vi "Corr Panel.vi"(8 "error in":errorcluster, 10 "adc session":T1={"niScope"={"channel cfg"=[], "sessions"=[], "multi cards"=FALSE, "channels"=0, "type"=enum."n/a", "memory [B/chn]"=0, "ext. clock [Hz]"=0.0, "samples count"=0, "use streaming"=FALSE, "proc setup"={"packet size [smpl]"=0, "current timeout [s]"=0.0, "blk2blk timeout [s]"=0.0, "event time"=timestamp(0 s since 1904-01-01), "temp sampl T [s]"=0.0, "data queue"=refnum, "stop notifier"=refnum, "proc ref"=refnum}, "sample width [B]"=0, "ranges [V]"=[], "trigger setup"={"coupling"=1, "level [V]"=0.0, "slope"=0, "mode"=enum."Immediate"}, "fs [Hz]"=0.0, "bitres [bit]"=0}, "3458A"={"channels"=[], "sync unit"={"VISA"="", "type"=enum."Picotest U6200A"}, "awg unit"={"type"=enum."Agilent 331xxA to 332xxA", "VISA"="", "enable 10MHz ref"=FALSE}, "sync mode"=enum."MASTER-SLAVE, MASTER clocked by TIMER", "streaming mode"=FALSE, "idn mode"=enum."Auto", "sampling mode"=enum."DCV", "Ts [s]"=0.0, "sample memory [B]"=0, "proc setup"={"channel id"=0, "packet size [smpl]"=0, "current timeout [s]"=0.0, "blk2blk timeout [s]"=0.0, "event time"=timestamp(0 s since 1904-01-01), "stop notifier"=refnum, "data queues"=[], "proc refs"=[], "bus semaphore"=refnum}, "sample size [B]"=0, "sample count"=0, "aux data"={"channel id"=0, "valid?"=[], "gain [V]"=[], "timestamp [s]"=[], "Ts [s]"=0.0, "abs timestamp"=timestamp(0 s since 1904-01-01), "t [deg C]"=[]}, "ranges [V]"=[], "aperture [s]"=0.0, "LEVEL trigger"={"edge"=enum."POS", "level [V]"=0.0, "coupling"=enum."DC"}, "trigger mode"=enum."AUTO", "measure temp.?"=FALSE, "disp mesages"=[], "shared bus?"=FALSE, "disable display?"=FALSE, "aper mode"=enum."Manual", "aper rules"=[]}, "dsdll"={"dsdll"={"dsdll path"=path "", "dsdll handle"=[], "output devices"=[], "capture devices"=[]}, "channels"=0, "device id"=0, "channel idns"=[], "proc setup"={"packet size [smpl]"=0, "current timeout [s]"=0.0, "blk2blk timeout [s]"=0.0, "event time"=timestamp(0 s since 1904-01-01), "data queue"=refnum, "stop notifier"=refnum, "proc ref"=refnum}, "samples count"=0, "fs [Hz]"=0.0}, "type"=enum."niScope", "channel idn str"=[], "aux instr idn str"=[], "modified?"=FALSE, "simadc"={"channels"=[], "range [V]"=0.0, "Ts step [s]"=0.0, "time [s]"=0.0, "fs [Hz]"=0.0, "count"=0, "smpl offset"=0, "set count"=0, "bit res"=0}, "force rst?"=FALSE, "exit mode"=enum."Immediate reset", "exit dly"=0.0, "exit tmr"=timestamp(0 s since 1904-01-01), "busy?"=FALSE, "accessed?"=FALSE, "QuADC session"={"channel cfg"=[], "sessions"=[], "multi cards"=FALSE, "channels"=0, "type"=enum."n/a", "memory [B/chn]"=0, "ext. clock [Hz]"=0.0, "samples count"=0, "use streaming"=FALSE, "proc setup"={"packet size [smpl]"=0, "current timeout [s]"=0.0, "blk2blk timeout [s]"=0.0, "event time"=timestamp(0 s since 1904-01-01), "temp sampl T [s]"=0.0, "data queue"=refnum, "stop notifier"=refnum, "proc ref"=refnum}, "sample width [B]"=0, "ranges [V]"=[], "trigger setup"={"coupling"=1, "level [V]"=0.0, "slope"=0, "mode"=enum."Immediate"}, "fs [Hz]"=0.0, "bitres [bit]"=0}} {"QuADC session"."trigger setup"."level [V]" format="%.2f"; "QuADC session"."trigger setup"."coupling" items=["AC"=0, "DC"=1, "HF Reject"=3, "LF Reject"=4, "AC Plus HF Reject"=1001]; "QuADC session"."channel cfg"."Clock fr. (Hz)" min=0.0 format="%#_9p"; "QuADC session"."channel cfg"."Number of JJ" min=1; "QuADC session"."channel cfg"."Range [Vpk]" min=0.0; "QuADC session"."channel cfg"."Channel" min=0; "3458A"."channels"."Range [Vpk]" min=0.0; "niScope"."trigger setup"."level [V]" format="%.2f"; "niScope"."trigger setup"."coupling" items=["AC"=0, "DC"=1, "HF Reject"=3, "LF Reject"=4, "AC Plus HF Reject"=1001]; "niScope"."channel cfg"."Range [Vpk]" min=0.0; "niScope"."channel cfg"."Channel" min=0}, 11 "transducers in":T45 {"transducers"."channels"."Phase index" min=1 step=1}) -> (0 "error out":errorcluster, 2 "adc session out":T1={"niScope"={"channel cfg"=[], "sessions"=[], "multi cards"=FALSE, "channels"=0, "type"=enum."n/a", "memory [B/chn]"=0, "ext. clock [Hz]"=0.0, "samples count"=0, "use streaming"=FALSE, "proc setup"={"packet size [smpl]"=0, "current timeout [s]"=0.0, "blk2blk timeout [s]"=0.0, "event time"=timestamp(0 s since 1904-01-01), "temp sampl T [s]"=0.0, "data queue"=refnum, "stop notifier"=refnum, "proc ref"=refnum}, "sample width [B]"=0, "ranges [V]"=[], "trigger setup"={"coupling"=1, "level [V]"=0.0, "slope"=0, "mode"=enum."Immediate"}, "fs [Hz]"=0.0, "bitres [bit]"=0}, "3458A"={"channels"=[], "sync unit"={"VISA"="", "type"=enum."Picotest U6200A"}, "awg unit"={"type"=enum."Agilent 331xxA to 332xxA", "VISA"="", "enable 10MHz ref"=FALSE}, "sync mode"=enum."MASTER-SLAVE, MASTER clocked by TIMER", "streaming mode"=FALSE, "idn mode"=enum."Auto", "sampling mode"=enum."DCV", "Ts [s]"=0.0, "sample memory [B]"=0, "proc setup"={"channel id"=0, "packet size [smpl]"=0, "current timeout [s]"=0.0, "blk2blk timeout [s]"=0.0, "event time"=timestamp(0 s since 1904-01-01), "stop notifier"=refnum, "data queues"=[], "proc refs"=[], "bus semaphore"=refnum}, "sample size [B]"=0, "sample count"=0, "aux data"={"channel id"=0, "valid?"=[], "gain [V]"=[], "timestamp [s]"=[], "Ts [s]"=0.0, "abs timestamp"=timestamp(0 s since 1904-01-01), "t [deg C]"=[]}, "ranges [V]"=[], "aperture [s]"=0.0, "LEVEL trigger"={"edge"=enum."POS", "level [V]"=0.0, "coupling"=enum."DC"}, "trigger mode"=enum."AUTO", "measure temp.?"=FALSE, "disp mesages"=[], "shared bus?"=FALSE, "disable display?"=FALSE, "aper mode"=enum."Manual", "aper rules"=[]}, "dsdll"={"dsdll"={"dsdll path"=path "", "dsdll handle"=[], "output devices"=[], "capture devices"=[]}, "channels"=0, "device id"=0, "channel idns"=[], "proc setup"={"packet size [smpl]"=0, "current timeout [s]"=0.0, "blk2blk timeout [s]"=0.0, "event time"=timestamp(0 s since 1904-01-01), "data queue"=refnum, "stop notifier"=refnum, "proc ref"=refnum}, "samples count"=0, "fs [Hz]"=0.0}, "type"=enum."niScope", "channel idn str"=[], "aux instr idn str"=[], "modified?"=FALSE, "simadc"={"channels"=[], "range [V]"=0.0, "Ts step [s]"=0.0, "time [s]"=0.0, "fs [Hz]"=0.0, "count"=0, "smpl offset"=0, "set count"=0, "bit res"=0}, "force rst?"=FALSE, "exit mode"=enum."Immediate reset", "exit dly"=0.0, "exit tmr"=timestamp(0 s since 1904-01-01), "busy?"=FALSE, "accessed?"=FALSE, "QuADC session"={"channel cfg"=[], "sessions"=[], "multi cards"=FALSE, "channels"=0, "type"=enum."n/a", "memory [B/chn]"=0, "ext. clock [Hz]"=0.0, "samples count"=0, "use streaming"=FALSE, "proc setup"={"packet size [smpl]"=0, "current timeout [s]"=0.0, "blk2blk timeout [s]"=0.0, "event time"=timestamp(0 s since 1904-01-01), "temp sampl T [s]"=0.0, "data queue"=refnum, "stop notifier"=refnum, "proc ref"=refnum}, "sample width [B]"=0, "ranges [V]"=[], "trigger setup"={"coupling"=1, "level [V]"=0.0, "slope"=0, "mode"=enum."Immediate"}, "fs [Hz]"=0.0, "bitres [bit]"=0}} {"QuADC session"."trigger setup"."level [V]" format="%.2f"; "QuADC session"."trigger setup"."coupling" items=["AC"=0, "DC"=1, "HF Reject"=3, "LF Reject"=4, "AC Plus HF Reject"=1001]; "QuADC session"."channel cfg"."Clock fr. (Hz)" min=0.0 format="%#_9p"; "QuADC session"."channel cfg"."Number of JJ" min=1; "QuADC session"."channel cfg"."Range [Vpk]" min=0.0; "QuADC session"."channel cfg"."Channel" min=0; "3458A"."channels"."Range [Vpk]" min=0.0; "niScope"."trigger setup"."level [V]" format="%.2f"; "niScope"."trigger setup"."coupling" items=["AC"=0, "DC"=1, "HF Reject"=3, "LF Reject"=4, "AC Plus HF Reject"=1001]; "niScope"."channel cfg"."Range [Vpk]" min=0.0; "niScope"."channel cfg"."Channel" min=0}, 3 "transducers out":T45 {"transducers"."channels"."Phase index" min=1 step=1})   [LabVIEW 2018]
doc: "Configuration panel for corrections."
uses:
  Corr Setup.ctl
  Corr Tranducer Item.ctl
  Corr Digitizers.ctl
  Corr Digitizer Channel.ctl
  adc/ADC Session.ctl
  drivers/niScope/niScope Session.ctl
  drivers/niScope/niScope Virtual Channel Config.ctl
  drivers/niScope/niScope Virtual Channel Mode.ctl
  drivers/niScope/niScope Virtual Channel Input Z.ctl
  drivers/niScope/niScope Virtual Channel Coupling.ctl
  drivers/niScope/niScope Type.ctl
  drivers/niScope/niScope Digitizing Process Options.ctl
  drivers/niScope/niScope Data Packet.ctl
  drivers/niScope/niScope Trigger Setup.ctl
  <instrlib>/niScope/Controls/niScope trigger coupling.ctl
  <instrlib>/niScope/Controls/niScope trigger slope.ctl
  drivers/DMM/3458A Digitizer Session.ctl
  drivers/DMM/3458A Virtual Channel Config.ctl
  drivers/Counter/Counter Session.ctl
  drivers/Counter/Counter Type.ctl
  drivers/AWG/AWG Session.ctl
  drivers/AWG/AWG Type.ctl
  drivers/DMM/3458A Sync Mode.ctl
  drivers/DMM/3458A Idn Mode.ctl
  drivers/DMM/3458A Digitizing Low Levels/Configure/Sampling Mode.ctl
  drivers/DMM/3458A Digitizing Process Options.ctl
  drivers/DMM/3458A Data Packet.ctl
  drivers/DMM/3458A Aux Record Data.ctl
  drivers/DMM/3458A Digitizing Low Levels/Configure/Level Setup.ctl
  drivers/DMM/3458A Digitizing Low Levels/Configure/First Sample Trigger.ctl
  drivers/DMM/3458A Aperture Selection Mode.ctl
  drivers/dsdll/DSDLL Session.ctl
  drivers/dsdll/dsdll source distribution/dsdll_instance.ctl
  drivers/dsdll/dsdll source distribution/dsdll_device_record.ctl
  drivers/dsdll/DSDLL Process Config.ctl
  drivers/dsdll/DSDLL Data Packet.ctl
  adc/ADC Type.ctl
  drivers/simulated_adc/SimAdc Config.ctl
  drivers/simulated_adc/SimAdc Channel Cfg.ctl
  adc/ADC On Close Action.ctl
  drivers/Quatsch_driver/QuADCDriver/QuADC Session.ctl
  drivers/Quatsch_driver/QuADCDriver/QuADC Virtual Channel Config.ctl
  drivers/Quatsch_driver/QuADCDriver/QuADC Virtual Channel Mode.ctl
  drivers/Quatsch_driver/QuADCDriver/QuADC Virtual Channel Input Z.ctl
  drivers/Quatsch_driver/QuADCDriver/QuADC Virtual Channel Coupling.ctl
  drivers/Quatsch_driver/QuADCDriver/QuADC Type.ctl
  drivers/Quatsch_driver/QuADCDriver/QuADC Digitizing Process Options.ctl
  drivers/Quatsch_driver/QuADCDriver/QuADC Data Packet.ctl
  drivers/Quatsch_driver/QuADCDriver/QuADC Trigger Setup.ctl
  varilib/SGUI Assign References Mode.ctl
  other/GUI Panel Control Action.ctl
  varilib/SGUI Assign Multiple Strings With Tags By Label.vi
  varilib/varilib.lvlib
  drivers/niScope/niScope Virtual Digitizer.lvlib
  drivers/DMM/3458A Virtual Digitizer.lvlib
  drivers/Counter/Counter.lvlib
  drivers/AWG/AWG.lvlib
  drivers/DMM/3458A Digitizing Low Levels/3458A Digitizing Low Levels.lvlib
  drivers/dsdll/DSDLL Virtual Digitizer.lvlib
  drivers/Quatsch_driver/QuADCDriver/QuADC Virtual Digitizer.lvlib
  drivers/dsdll/dsdll source distribution/dsdll.lvlib
panel:
  in  "tc corr":enum32{"Transducers", "Digitizers"}(tab)
  in  "trans list":T43(array[cluster]) caption="List of the transducers" {"Phase index" min=1 step=1; "chn lo" items=["Not used"]}
  out "dig corr stat":string caption="Correction status"
  in  "btn check dig":bool
  in  "btn reload dig":bool
  in  "btn clear dig":bool
  out "dig corr chns":T44[](array[typedef]) caption="Correction channels"
  out "dig corr path":string caption="Correction file path"
  out "dig corr name":string caption="Correction name"
  in  "btn open dig":bool
  out "status":string caption="Status"
  in  "btn cancel":bool
  in  "btn ok":bool
  # "IP Address"
  # "."
  # "."
  # "."
  # ":"
  # "IP Address"
  # "."
  # "."
  # "."
  # ":"
  # "ADC:"
  # "ADC:"
  # "ADC:"
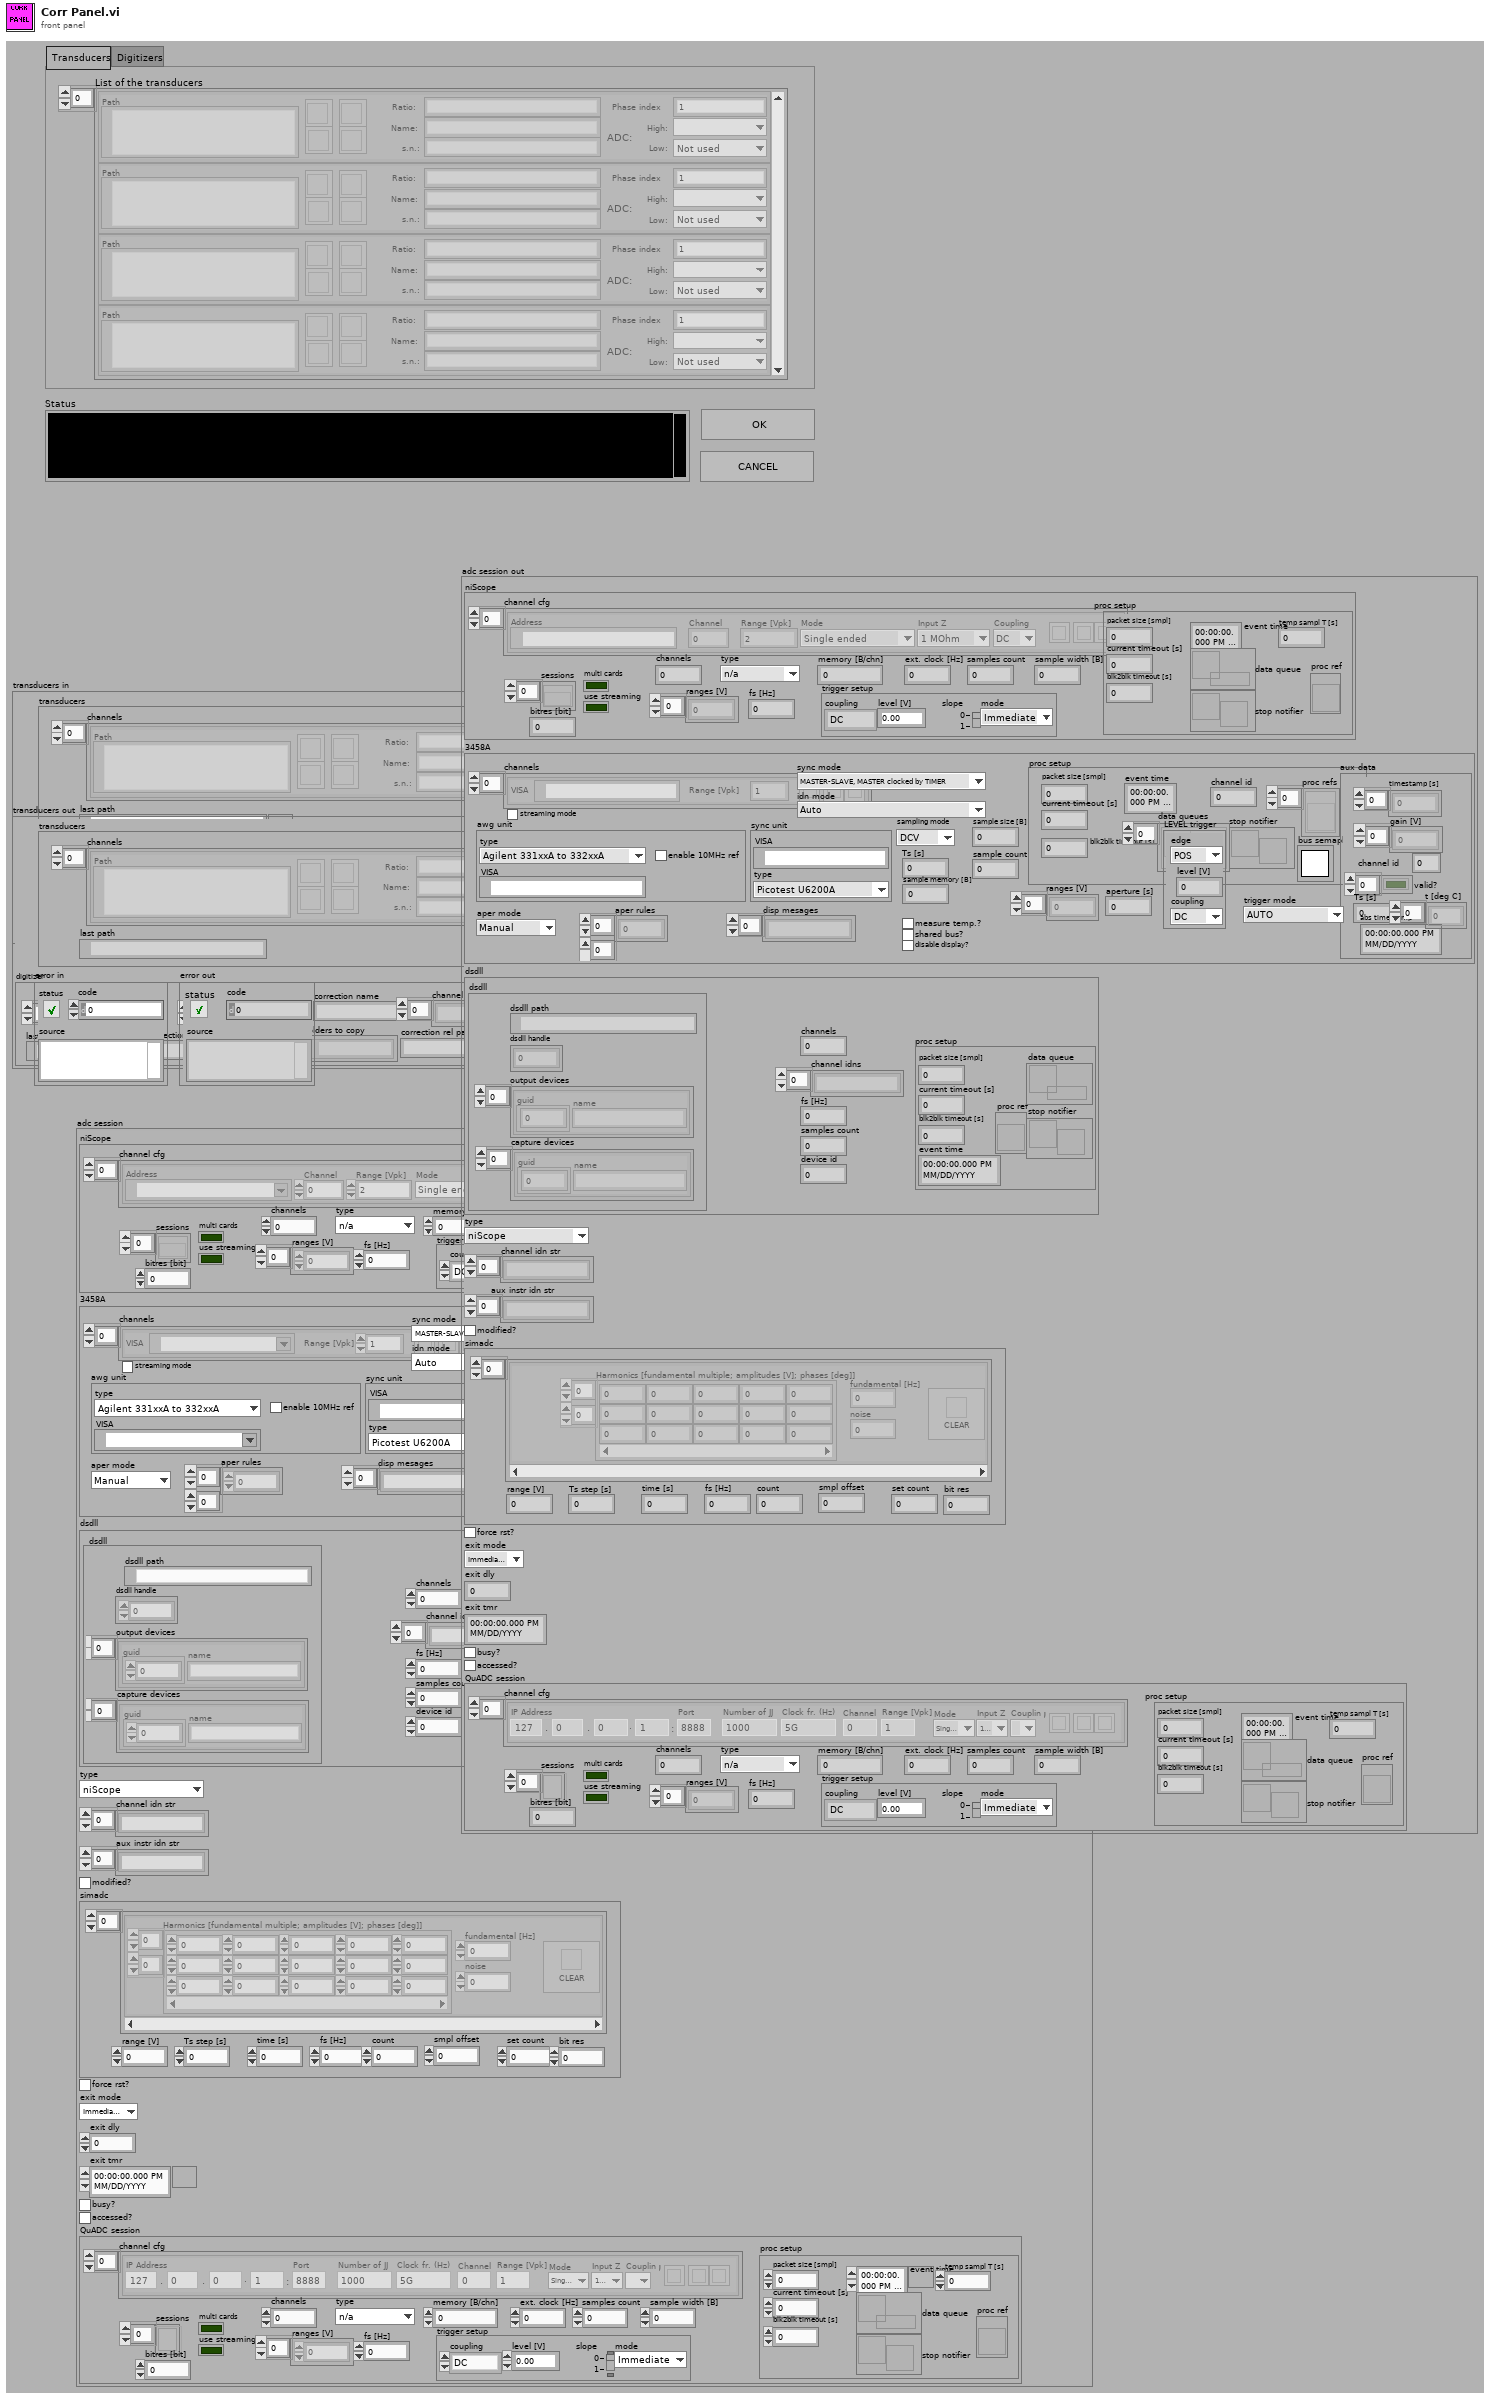
[diagram p1: front panel]
types:
  T1 = typedef "ADC Session.ctl" = cluster{"niScope":T2, "3458A":T12, "dsdll":T27, "type":T31, "channel idn str":string[], "aux instr idn str":string[], "modified?":bool, "simadc":T32, "force rst?":bool, "exit mode":T34, "exit dly":dbl, "exit tmr":timestamp, "busy?":bool, "accessed?":bool, "QuADC session":T35}
  T2 = typedef "niScope Virtual Digitizer.lvlib/niScope Session.ctl" = cluster{"channel cfg":T3[], "sessions":refnum<k20>[], "multi cards":bool, "channels":i32, "type":T7, "memory [B/chn]":i32, "ext. clock [Hz]":dbl, "samples count":i64, "use streaming":bool, "proc setup":T8, "sample width [B]":i32, "ranges [V]":dbl[], "trigger setup":T9, "fs [Hz]":dbl, "bitres [bit]":i32}
  T3 = typedef "niScope Virtual Digitizer.lvlib/niScope Virtual Channel Config.ctl" = cluster{"Address":refnum<k15>, "Channel":i32, "Mode":T4, "Input Z":T5, "Coupling":T6, "Range [Vpk]":dbl, "btn clr":bool, "btn up":bool, "btn down":bool}
  T4 = typedef "niScope Virtual Digitizer.lvlib/niScope Virtual Channel Mode.ctl" = enum16{"Single ended", "Unbal. differential", "Differential"}
  T5 = typedef "niScope Virtual Digitizer.lvlib/niScope Virtual Channel Input Z.ctl" = enum16{"1 MOhm", "50 Ohm"}
  T6 = typedef "niScope Virtual Digitizer.lvlib/niScope Virtual Channel Coupling.ctl" = enum16{"AC", "DC", "GND"}
  T7 = typedef "niScope Virtual Digitizer.lvlib/niScope Type.ctl" = enum16{"n/a", "5922"}
  T8 = typedef "niScope Virtual Digitizer.lvlib/niScope Digitizing Process Options.ctl" = cluster{"packet size [smpl]":i64, "current timeout [s]":dbl, "blk2blk timeout [s]":dbl, "event time":timestamp, "temp sampl T [s]":dbl, "data queue":refnum<queue>, "stop notifier":refnum<notifier>, "proc ref":refnum<vi>}
  T9 = typedef "niScope Virtual Digitizer.lvlib/niScope Trigger Setup.ctl" = cluster{"coupling":T10, "level [V]":dbl, "slope":T11, "mode":enum16{"Immediate", "External", "Level"}}
  T10 = typedef "niScope trigger coupling.ctl" = u16
  T11 = typedef "niScope trigger slope.ctl" = i32
  T12 = typedef "3458A Virtual Digitizer.lvlib/3458A Digitizer Session.ctl" = cluster{"channels":T13[], "sync unit":T14, "awg unit":T16, "sync mode":T18, "streaming mode":bool, "idn mode":T19, "sampling mode":T20, "Ts [s]":dbl, "sample memory [B]":i32, "proc setup":T21, "sample size [B]":i32, "sample count":i32, "aux data":T23, "ranges [V]":dbl[], "aperture [s]":dbl, "LEVEL trigger":T24, "trigger mode":T25, "measure temp.?":bool, "disp mesages":string[], "shared bus?":bool, "disable display?":bool, "aper mode":T26, "aper rules":dbl[][]}
  T13 = typedef "3458A Virtual Digitizer.lvlib/3458A Virtual Channel Config.ctl" = cluster{"VISA":refnum<visa-resource-name>, "Range [Vpk]":dbl, "btn clr":bool, "btn up":bool, "btn down":bool}
  T14 = typedef "Counter.lvlib/Counter Session.ctl" = cluster{"VISA":refnum<visa-resource-name>, "type":T15}
  T15 = typedef "Counter.lvlib/Counter Type.ctl" = enum16{"Picotest U6200A", "dummy"}
  T16 = typedef "AWG.lvlib/AWG Session.ctl" = cluster{"type":T17, "VISA":refnum<visa-resource-name>, "enable 10MHz ref":bool}
  T17 = typedef "AWG.lvlib/AWG Type.ctl" = enum16{"Agilent 331xxA to 332xxA", "Agilent 335xxA to 336xxA", "Tektronix AFG3101C", "dummy"}
  T18 = typedef "3458A Virtual Digitizer.lvlib/3458A Sync Mode.ctl" = enum16{"MASTER-SLAVE, MASTER clocked by TIMER", "MASTER-SLAVE, MASTER clocked by AWG", "ALL clocked by AWG", "MASTER-SLAVE, ALL clocked by TIMER", "ALL clocked by AWG with DFLL"}
  T19 = typedef "3458A Virtual Digitizer.lvlib/3458A Idn Mode.ctl" = enum16{"Auto", "Sequential (chn A, chn B, ...)", "From calibration string"}
  T20 = typedef "3458A Virtual Digitizer.lvlib/3458A Digitizing Low Levels.lvlib/Sampling Mode.ctl" = enum16{"DCV", "DSDC", "DSAC"}
  T21 = typedef "3458A Virtual Digitizer.lvlib/3458A Digitizing Process Options.ctl" = cluster{"channel id":i32, "packet size [smpl]":i32, "current timeout [s]":dbl, "blk2blk timeout [s]":dbl, "event time":timestamp, "stop notifier":refnum<notifier>, "data queues":refnum<queue>[], "proc refs":refnum<vi>[], "bus semaphore":T22}
  T22 = typedef "Semaphore RefNum" = refnum<k1>
  T23 = typedef "3458A Virtual Digitizer.lvlib/3458A Aux Record Data.ctl" = cluster{"channel id":i32, "valid?":bool[], "gain [V]":dbl[], "timestamp [s]":dbl[], "Ts [s]":dbl, "abs timestamp":timestamp, "t [deg C]":dbl[]}
  T24 = typedef "3458A Virtual Digitizer.lvlib/3458A Digitizing Low Levels.lvlib/Level Setup.ctl" = cluster{"edge":enum16{"POS", "NEG"}, "level [V]":dbl, "coupling":enum16{"DC", "AC"}}
  T25 = typedef "3458A Virtual Digitizer.lvlib/3458A Digitizing Low Levels.lvlib/First Sample Trigger.ctl" = enum16{"AUTO", "EXT", "SYN", "SGL", "HOLD", "LEVEL"}
  T26 = typedef "3458A Virtual Digitizer.lvlib/3458A Aperture Selection Mode.ctl" = enum16{"Manual", "Maximum", "Table"}
  T27 = typedef "DSDLL Virtual Digitizer.lvlib/DSDLL Session.ctl" = cluster{"dsdll":T28, "channels":i32, "device id":i32, "channel idns":string[], "proc setup":T30, "samples count":i32, "fs [Hz]":dbl}
  T28 = typedef "dsdll.lvlib/dsdll_instance.ctl" = cluster{"dsdll path":path, "dsdll handle":u8[], "output devices":T29[], "capture devices":T29[]}
  T29 = typedef "dsdll.lvlib/dsdll_device_record.ctl" = cluster{"guid":u8[], "name":string}
  T30 = typedef "DSDLL Virtual Digitizer.lvlib/DSDLL Process Config.ctl" = cluster{"packet size [smpl]":i32, "current timeout [s]":dbl, "blk2blk timeout [s]":dbl, "event time":timestamp, "data queue":refnum<queue>, "stop notifier":refnum<notifier>, "proc ref":refnum<vi>}
  T31 = typedef "ADC Type.ctl" = enum16{"niScope", "3458A", "DirectSound DLL", "dummy", "QuADC"}
  T32 = typedef "SimAdc Config.ctl" = cluster{"channels":T33[], "range [V]":dbl, "Ts step [s]":dbl, "time [s]":dbl, "fs [Hz]":dbl, "count":i64, "smpl offset":i64, "set count":i64, "bit res":i32}
  T33 = typedef "SimAdc Channel Cfg.ctl" = cluster{"harmonics":dbl[][], "btn clear":bool, "noise":dbl, "fundamental [Hz]":dbl}
  T34 = typedef "ADC On Close Action.ctl" = enum16{"Immediate reset", "Delayed reset"}
  T35 = typedef "QuADC Virtual Digitizer.lvlib/QuADC Session.ctl" = cluster{"channel cfg":T36[], "sessions":refnum<k5>[], "multi cards":bool, "channels":i32, "type":T40, "memory [B/chn]":i32, "ext. clock [Hz]":dbl, "samples count":i64, "use streaming":bool, "proc setup":T41, "sample width [B]":i32, "ranges [V]":dbl[], "trigger setup":T42, "fs [Hz]":dbl, "bitres [bit]":i32}
  T36 = typedef "QuADC Virtual Digitizer.lvlib/QuADC Virtual Channel Config.ctl" = cluster{"Channel":i32, "Mode":T37, "Input Z":T38, "Coupling":T39, "Range [Vpk]":dbl, "btn clr":bool, "btn up":bool, "btn down":bool, "IP address A":u8, "IP address B":u8, "IP address C":u8, "IP address D":u8, "Port":u16, "Number of JJ":u32, "Clock fr. (Hz)":dbl}
  T37 = typedef "QuADC Virtual Digitizer.lvlib/QuADC Virtual Channel Mode.ctl" = enum16{"Single ended", "Unbal. differential", "Differential"}
  T38 = typedef "QuADC Virtual Digitizer.lvlib/QuADC Virtual Channel Input Z.ctl" = enum16{"1 MOhm", "50 Ohm"}
  T39 = typedef "QuADC Virtual Digitizer.lvlib/QuADC Virtual Channel Coupling.ctl" = enum16{"AC", "DC", "GND"}
  T40 = typedef "QuADC Virtual Digitizer.lvlib/QuADC Type.ctl" = enum16{"n/a", "v1"}
  T41 = typedef "QuADC Virtual Digitizer.lvlib/QuADC Digitizing Process Options.ctl" = cluster{"packet size [smpl]":i64, "current timeout [s]":dbl, "blk2blk timeout [s]":dbl, "event time":timestamp, "temp sampl T [s]":dbl, "data queue":refnum<queue>, "stop notifier":refnum<notifier>, "proc ref":refnum<vi>}
  T42 = typedef "QuADC Virtual Digitizer.lvlib/QuADC Trigger Setup.ctl" = cluster{"coupling":T10, "level [V]":dbl, "slope":T11, "mode":enum16{"Immediate", "External", "Level"}}
  T43 = cluster{"Path":path, "Ratio:":string, "Name:":string, "btn rem":bool, "btn up":bool, "btn down":bool, "s.n.:":string, "btn open":bool, "ratio o/i":dbl, "chn hi":u16, "chn lo":u16, "Phase index":i32}[]
  T44 = typedef "Corr Digitizer Channel.ctl" = cluster{"Correction identifier":string, "Channel correction file ok?":bool, "Channel matches digitizer HW?":bool, "Correction channel name":string, "HW channel identifier":string}
  T45 = typedef "Corr Setup.ctl" = cluster{"transducers":cluster{"channels":T46[], "last path":path}, "digitizer":T47}
  T46 = typedef "Corr Tranducer Item.ctl" = cluster{"Path":path, "Ratio:":string, "Name:":string, "btn rem":bool, "btn up":bool, "btn down":bool, "s.n.:":string, "btn open":bool, "ratio o/i":dbl, "chn hi":u16, "chn lo":u16, "Phase index":i32}
  T47 = typedef "Corr Digitizers.ctl" = cluster{"last path":path, "channel paths":path[], "channel idns":string[], "correction name":string, "channel names":string[], "folders to copy":path[], "channel valid":bool[], "correction path":path, "correction rel path":string, "rel folders to copy":string[]}
  T48 = typedef "GUI Panel Control Action.ctl" = enum16{"Open panel", "Close panel", "Bring To Front"}
  T49 = typedef "varilib.lvlib/SGUI Assign References Mode.ctl" = enum16{"Add to stack", "Overwrite", "Release last", "Release ID"}
  T50 = cluster{"Path":path, "Ratio:":string, "Name:":string, "btn rem":bool, "btn up":bool, "btn down":bool, "s.n.:":string, "btn open":bool, "ratio o/i":dbl, "chn hi":u16, "chn lo":u16, "Phase index":i32}
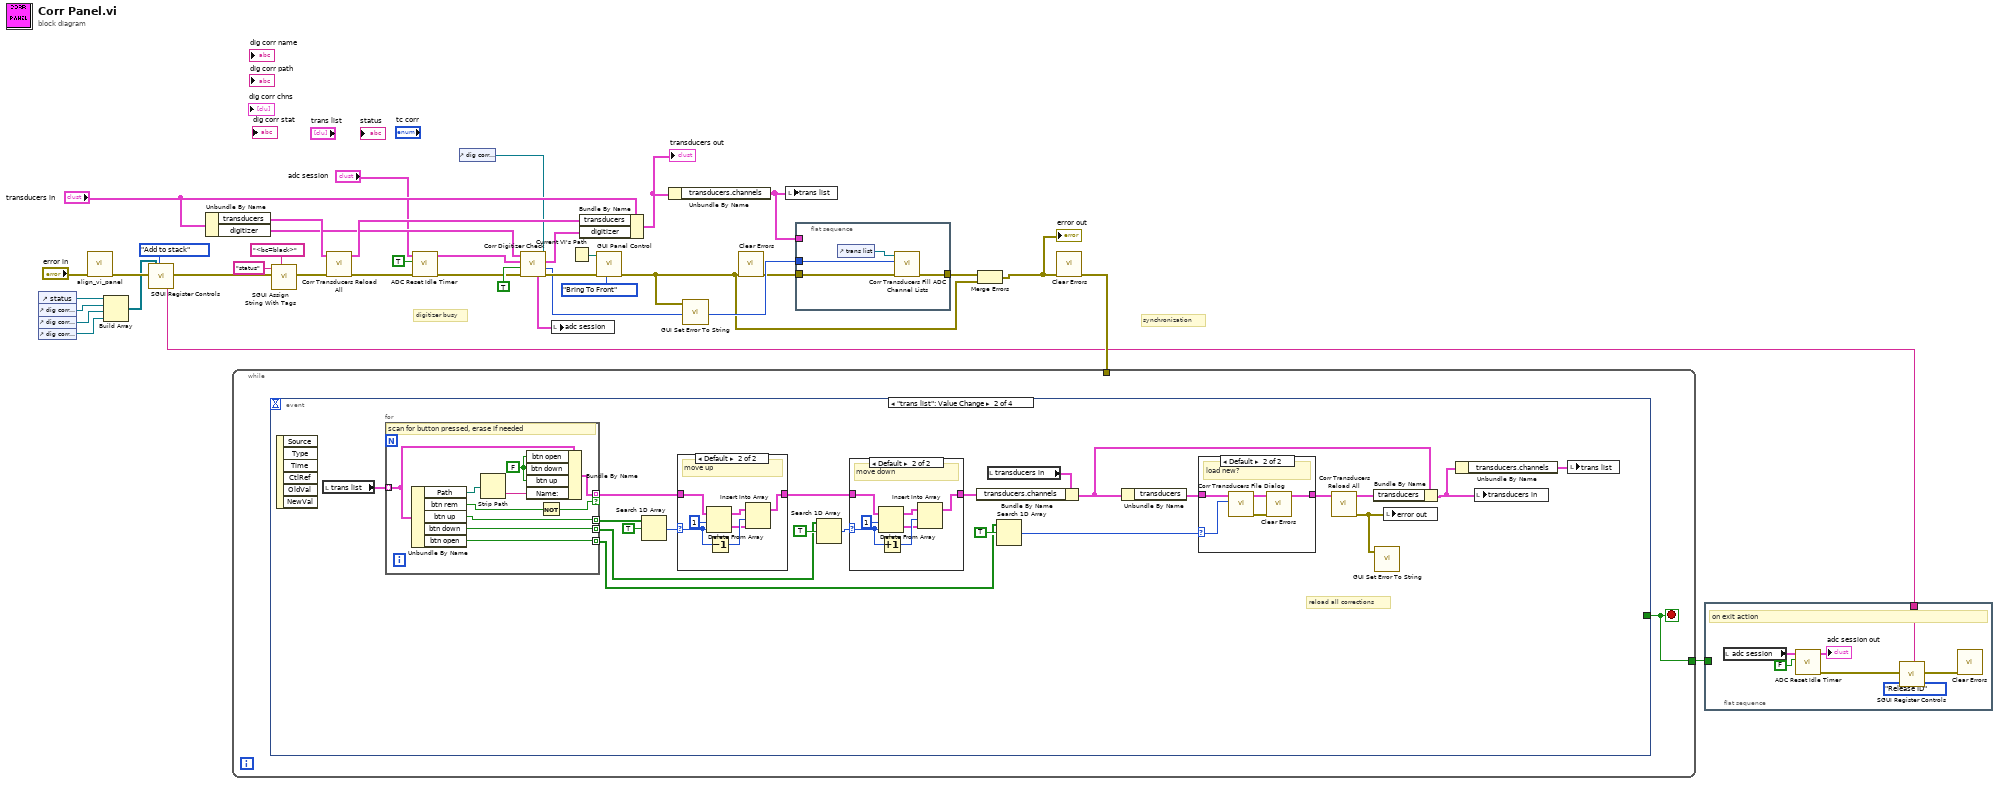
[diagram p0: block diagram]
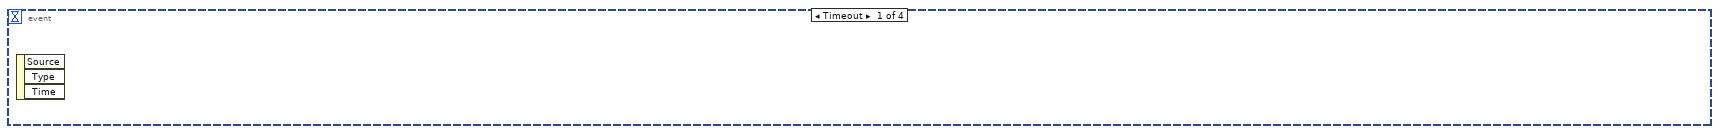
[diagram p2: hidden frame]
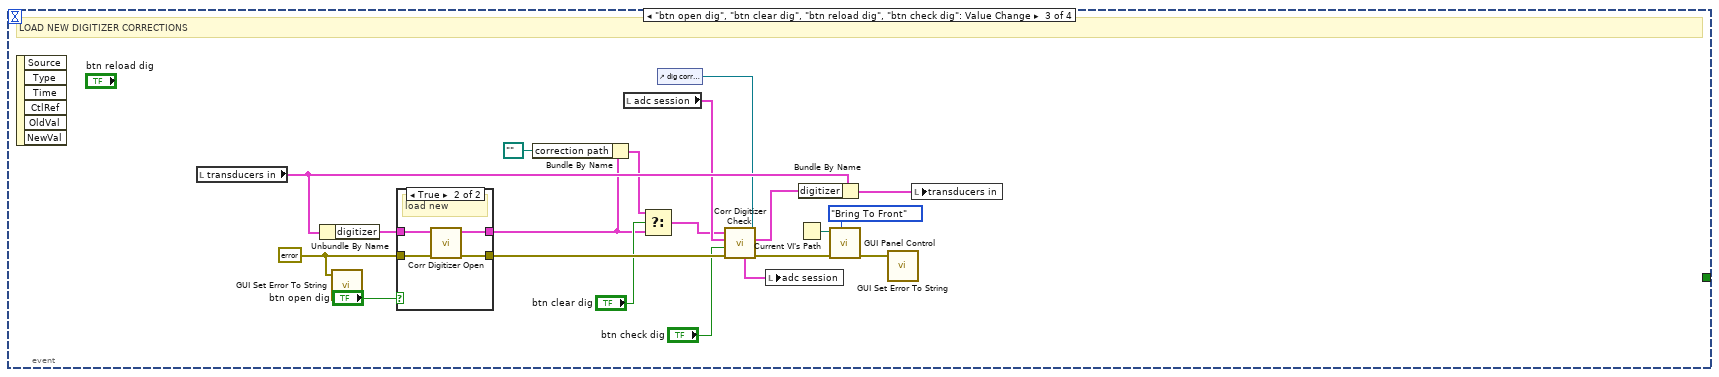
[diagram p6: hidden frame]
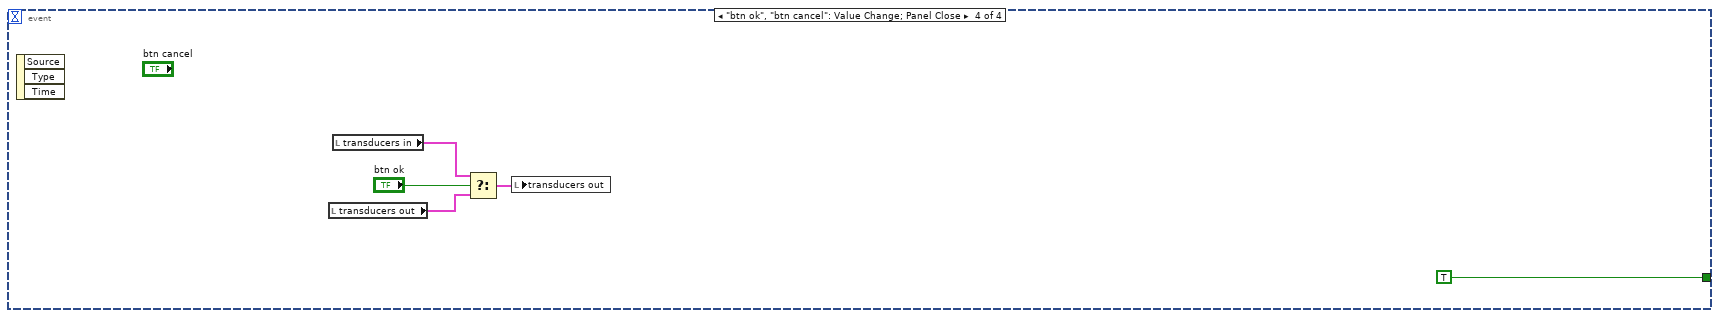
[diagram p8: hidden frame]
diagram:
  # "digitizer busy"
  # "synchronization"
  n1 = control-ref of="status"() -> (w24:refnum<vi>)
  n2 = control-ref of="dig corr name"() -> (w23:refnum<vi>)
  n3 = control-ref of="dig corr path"() -> (w22:refnum<vi>)
  n4 = control-ref of="dig corr stat"() -> (w21:refnum<vi>)
  n5 = call "align_vi_panel.vi"("error in"="error in") -> ("error out"=w38:errorcluster)  [unwired: 10 in]
  n6 = Build Array(w24, w23, w22, w21) -> (w25:refnum<vi>[])
  n7 = call "SGUI Register Controls.vi"("error in"=w38, "control references (empty)"=w25, "register mode (overwrite)"=SGUI_Assign_References_Mode."Add to stack") -> ("assigned ID"=w7:string, "error out"=w35:errorcluster)  [unwired: 14 in, 1 out]
  n8 = Unbundle By Name("transducers in") -> ("transducers"=w29:cluster{"channels":T46[], "last path":path}, "digitizer"=w19:T47)
  n9 = call-poly "SGUI Assign String With Tags.vi"("error in"=w35, "label(s) (empty)"="status", "string (empty)"="<bc=black>") -> ("error out"=w30:errorcluster)  [unwired: 7 in, 1 out]
  n10 = call "Corr Transducers Reload All.vi"("error in"=w30, "transducers in"=w29) -> ("error out"=w6:errorcluster, "transducers out"=w27:cluster{"channels":T46[], "last path":path})  [unwired: 8 in]
  n11 = call "ADC Reset Idle Timer.vi"("error in"=w6, "set busy (False)"=TRUE, "adc session in"="adc session") -> ("error out"=w4:errorcluster, "adc session out"=w2:T1)  [unwired: 7 in]
  n12 = control-ref of="dig corr chns"() -> (w17:refnum<vi>)
  n13 = call "Corr Digitizer Check.vi"("dig corr chns ref"=w17, "error in"=w4, "check HW? (False)"=TRUE, "adc session"=w2, "digitizer corrections in"=w19) -> ("error out"=w16:errorcluster, "adc chan. count"=w12:i32, "digitizer corrections out"=w20:T47, "adc session out"=w1:T1)  [unwired: 3 in]
  n14 = local write "adc session"(w1) -> ()
  n15 = Current VI's Path() -> (path=w15:path)
  n16 = Bundle By Name(cluster="transducers in", "transducers"=w27, "digitizer"=w20) -> (w26:T45)
  "transducers out" <- w26
  n17 = call "GUI Panel Control.vi"("action (open panel)"=GUI_Panel_Control_Action."Bring To Front", "error in (no error)"=w16, "vi path"=w15) -> ("error out"=w9:errorcluster)  [unwired: 8 in]
  n18 = Unbundle By Name(w26) -> ("transducers.channels"=w13:T46[])
  n19 = call "GUI Set Error To String.vi"("error in (no error)"=w9) -> ()  [unwired: 4 in]
  n20 = call <vilib>:"Clear Errors.vi"("error in (no error)"=w9) -> ("error out"=w11:errorcluster)  [unwired: 5 in, 1 out]
  n21 = local write "trans list"(w13) -> ()
  n22 = flat-sequence {
    tunnel: w11 -> [w42]
    tunnel: [w41] -> w10
    tunnel: w13 -> [_]
    tunnel: w12 -> [w40]
    frame #0 {
      n23 = control-ref of="trans list"() -> (w39:refnum<vi>)
      n24 = call "Corr Transducers Fill ADC Channel Lists.vi"("error in"=w42, "digitizer channels count (0)"=w40, "transducer list ref"=w39) -> ("error out"=w41:errorcluster)  [unwired: 7 in, 1 out]
    }
  }
  n25 = Merge Errors(w10, w9) -> (w8:errorcluster)
  "error out" <- w8
  n26 = call <vilib>:"Clear Errors.vi"("error in (no error)"=w8) -> ("error out"=w32:errorcluster)  [unwired: 5 in, 1 out]
  n27 = while {
    tunnel: w32 -> [_]
    tunnel: [w43] -> w31
    stop <- w43 stop-if-true
    n28 = event shown="[1] \"trans list\": Value Change" {
      selector: _ -> [_ _ _ _]
      dyn-events: _ -> [_ _ _ _]
      timeout: _ -> [_ _ _ _]
      tunnel: [_ _ _ TRUE] -> w43
      event Timeout {
        n29 = event-data() -> ()  [unwired: 1 in, 3 out]
      }
      event "trans list": Value Change {
        # "reload all corrections"
        n30 = event-data() -> ()  [unwired: 1 in, 6 out]
        n31 = local read "trans list"() -> (w56:T43)
        n32 = for {
          tunnel: w56 -> [w94] mode=indexing
          tunnel: [w92] -> w62 mode=indexing if=w90
          tunnel: [w89] -> w64 mode=indexing
          tunnel: [w88] -> w57 mode=indexing
          tunnel: [w86] -> w54 mode=indexing
          w87 = FALSE ("btn down")
          # "scan for button pressed, erase if needed"
          n33 = Unbundle By Name(w94) -> ("Path"=w95:path, "btn rem"=w91:bool, "btn up"=w89:bool, "btn down"=w88:bool, "btn open"=w86:bool)
          n34 = Strip Path(path=w95) -> (name=w93:string)  [unwired: 1 out]
          n35 = Bundle By Name(cluster=w94, "btn open"=w87, "btn down"=w87, "btn up"=w87, "Name:"=w93) -> (w92:T50)
          n36 = Not(x=w91) -> (.not. x?=w90:bool)
        }
        n37 = Search 1D Array(1D array=w64, element=TRUE) -> (index of element=w61:i32)  [unwired: 1 in]
        n38 = case shown="Default" w61 {
          selector: w61 -> [_ w83]
          tunnel: w62 -> [w78 w81]
          tunnel: [w78 w82] -> w58
          frame -1, 0 {
          }
          frame Default {
            # "move up"
            n39 = Delete From Array(array=w81, length=1, index=w83) -> (deleted portion=w79:T43, array with subset deleted=w80:T43)
            n40 = Decrement(x=w83) -> (x-1=w84:i32)
            n41 = Insert Into Array(array=w80, index=w84, new element=w79) -> (w82:T43)
          }
        }
        n42 = Search 1D Array(1D array=w57, element=TRUE) -> (index of element=w59:i32)  [unwired: 1 in]
        n43 = case shown="Default" w59 {
          selector: w59 -> [_ w73]
          tunnel: w58 -> [w70 w77]
          tunnel: [w70 w72] -> w52
          frame -1 {
          }
          frame Default {
            # "move down"
            n44 = Delete From Array(array=w77, length=1, index=w73) -> (deleted portion=w71:T43, array with subset deleted=w76:T43)
            n45 = Increment(x=w73) -> (x+1=w74:i32)
            n46 = Insert Into Array(array=w76, index=w74, new element=w71) -> (w72:T43)
          }
        }
        n47 = local read "transducers in"() -> (w53:T45)
        n48 = Bundle By Name(cluster=w53, "transducers.channels"=w52) -> (w46:T45)
        n49 = Search 1D Array(1D array=w54, element=TRUE) -> (index of element=w51:i32)  [unwired: 1 in]
        n50 = Unbundle By Name(w46) -> ("transducers"=w47:cluster{"channels":T46[], "last path":path})
        n51 = case shown="Default" w51 {
          selector: w51 -> [_ w66]
          tunnel: w47 -> [w65 w69]
          tunnel: [w65 w67] -> w50
          frame -1 {
          }
          frame Default {
            # "load new?"
            n52 = call "Corr Transducers File Dialog.vi"("channel index (0)"=w66, "transducers in"=w69) -> ("error out"=w68:errorcluster, "transducers out"=w67:cluster{"channels":T46[], "last path":path})  [unwired: 8 in]
            n53 = call <vilib>:"Clear Errors.vi"("error in (no error)"=w68) -> ()  [unwired: 5 in, 2 out]
          }
        }
        n54 = call "Corr Transducers Reload All.vi"("transducers in"=w50) -> ("error out"=w48:errorcluster, "transducers out"=w45:cluster{"channels":T46[], "last path":path})  [unwired: 9 in]
        n55 = Bundle By Name(cluster=w46, "transducers"=w45) -> (w44:T45)
        n56 = call "GUI Set Error To String.vi"("error in (no error)"=w48) -> ()  [unwired: 4 in]
        n57 = local write "error out"(w48) -> ()
        n58 = Unbundle By Name(w44) -> ("transducers.channels"=w49:T46[])
        n59 = local write "transducers in"(w44) -> ()
        n60 = local write "trans list"(w49) -> ()
      }
      event "btn open dig", "btn clear dig", "btn reload dig", "btn check dig": Value Change {
        w112 = errorcluster {"status"=FALSE, "code"=0, "source"=""} ("error in")
        # "LOAD NEW DIGITIZER CORRECTIONS"
        n61 = event-data() -> ()  [unwired: 1 in, 6 out]
        n62 = local read "transducers in"() -> (w114:T45)
        n63 = Unbundle By Name(w114) -> ("digitizer"=w115:T47)
        n64 = call "GUI Set Error To String.vi"("error in (no error)"=w112) -> ()  [unwired: 4 in]
        n65 = case shown="True" "btn open dig" {
          tunnel: w115 -> [w116 w121]
          tunnel: w112 -> [w117 w120]
          tunnel: [w117 w119] -> w111
          tunnel: [w116 w118] -> w105
          frame False {
          }
          frame True {
            # "load new"
            n66 = call "Corr Digitizer Open.vi"("error in"=w120, "digitizer corrections in"=w121) -> ("error out"=w119:errorcluster, "digitizer corrections out"=w118:T47)  [unwired: 6 in, 2 out]
          }
        }
        n67 = Bundle By Name(cluster=w105, "correction path"=path "") -> (w104:T47)
        n68 = local read "adc session"() -> (w110:T1)
        n69 = Select(t=w104, s="btn clear dig", f=w105) -> (s? t:f=w107:T47)
        n70 = control-ref of="dig corr chns"() -> (w109:refnum<vi>)
        n71 = call "Corr Digitizer Check.vi"("dig corr chns ref"=w109, "error in"=w111, "check HW? (False)"="btn check dig", "adc session"=w110, "digitizer corrections in"=w107) -> ("error out"=w99:errorcluster, "digitizer corrections out"=w102:T47, "adc session out"=w96:T1)  [unwired: 3 in, 1 out]
        n72 = local write "adc session"(w96) -> ()
        n73 = Current VI's Path() -> (path=w100:path)
        n74 = Bundle By Name(cluster=w114, "digitizer"=w102) -> (w113:T45)
        n75 = call "GUI Panel Control.vi"("action (open panel)"=GUI_Panel_Control_Action."Bring To Front", "error in (no error)"=w99, "vi path"=w100) -> ("error out"=w98:errorcluster)  [unwired: 8 in]
        n76 = call "GUI Set Error To String.vi"("error in (no error)"=w98) -> ()  [unwired: 4 in]
        n77 = local write "transducers in"(w113) -> ()
      }
      event "btn ok", "btn cancel": Value Change; Panel Close {
        n78 = event-data() -> ()  [unwired: 1 in, 3 out]
        n79 = local read "transducers out"() -> (w122:T45)
        n80 = local read "transducers in"() -> (w124:T45)
        n81 = Select(t=w124, s="btn ok", f=w122) -> (s? t:f=w123:T45)
        n82 = local write "transducers out"(w123) -> ()
      }
    }
  }
  n83 = flat-sequence {
    tunnel: w31 -> [_]
    tunnel: w7 -> [w131]
    frame #0 {
      # "on exit action"
      n84 = local read "adc session"() -> (w129:T1)
      n85 = call "ADC Reset Idle Timer.vi"("set busy (False)"=FALSE, "adc session in"=w129) -> ("error out"=w130:errorcluster, "adc session out"=→"adc session out":T1)  [unwired: 8 in]
      n86 = call "SGUI Register Controls.vi"("error in"=w130, "register mode (overwrite)"=SGUI_Assign_References_Mode."Release ID", "controls ID (empty)"=w131) -> ("error out"=w132:errorcluster)  [unwired: 14 in, 2 out]
      n87 = call <vilib>:"Clear Errors.vi"("error in (no error)"=w132) -> ()  [unwired: 5 in, 2 out]
    }
  }
